vi "Recognize Text (Greyscale).vi"(8 "error in (no error)":errorcluster, 10 "Greyscale Image in":T1, 11 "Text Recognizer in":refnum<class "Text Recognizer.lvclass">) -> (0 "error out":errorcluster, 2 "Recognition":string, 3 "Text Recognizer":refnum<class "Text Recognizer.lvclass">)   [LabVIEW 2020, in "feature_detection.lvlib" / "Text Recognizer.lvclass"]
uses:
  Text Recognizer.lvclass
  Text Recognizer.lvclass/Text Recognizer.ctl
  2becd383-3adf-4b47-81eb-e38e0ef2f6e5.vi
  image/Greyscale Image.ctl
  image/image.lvlib
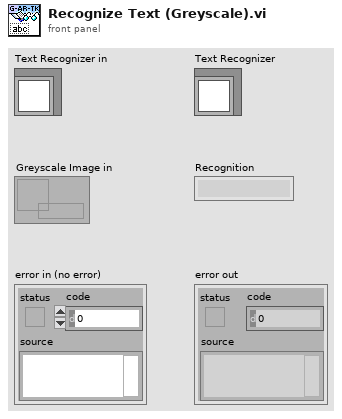
[diagram p1: front panel]
types:
  T1 = typedef "image.lvlib/Greyscale Image.ctl" = refnum<data-value>
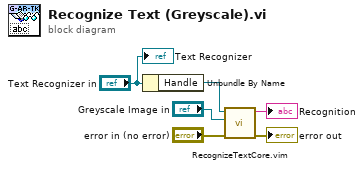
[diagram p0: block diagram]
diagram:
  n1 = Unbundle By Name("Text Recognizer in") -> ("Handle"=w4:refnum<data-value>)
  n2 = call "RecognizeTextCore.vim"("error in (no error)"="error in (no error)", "ARGB Image in"="Greyscale Image in", "Data Value Reference in"=w4) -> ("error out"=→"error out":errorcluster, "Recognition"=→"Recognition":string)  [unwired: 7 in]
  "Text Recognizer" <- "Text Recognizer in"
